vi "[FPGA] DeltaSig Main.vi"() -> ()   [LabVIEW 2015]
doc: "This VI provides a template for customizing a waveform acquisition using delta-sigma based NI C Series analog input smodules."
uses:
  <vilib>/rvi/Emulation/niFpgaGetClockAttributes.vi
  <vilib>/rvi/Emulation/niFpgaSctlEmulationGetInTimedLoop.vi
  <vilib>/rvi/Emulation/niFpgaEmulationReportErrorSimple.vi
  <vilib>/LabVIEW Targets/FPGA/cRIO/shared/nicrio_DsaDataRateApi/_nicrio_9234GetDataRate131.vi
  <vilib>/rvi/Emulation/niFpgaProcessEmulError.vi
  <vilib>/rvi/eio/common/nirviEmuTemplatePropertySet_errors.vi
  <vilib>/rvi/eio/common/nirviEmuTemplateMethod_errors.vi
  <vilib>/rvi/interface/RandomDataEmulation/niFpgaRandomDataHandleErrors.vi
  <vilib>/rvi/Emulation/niFpgaCriticalErrorInLSC.vi
  <vilib>/eio/EIOPropertyNode/EIOPropertyNode.xnode
  <vilib>/LabVIEW Targets/FPGA/cRIO/shared/nicrio_ModuleControls/nicrio_cRIO-9234_DataRatesRing2.ctl
  <vilib>/eio/EIONode/EIONode.xnode
  <vilib>/rvi/DataTransferAndStorage/Container/XNode/niFpgaContainer.xnode
  <vilib>/rvi/interface/RandomDataEmulation/nirviRandomDataFpgaReadWriteTemplate.vi
  <vilib>/rvi/eio/common/nirviEmuTemplatePropertyGet_errors.vi
  <vilib>/rvi/eio/common/nirviEmuTemplatePropertyGet_noerrors.vi
  <vilib>/rvi/eio/common/nirviEmuTemplatePropertySet_noerrors.vi
panel:
  out "oclk freq":u32
  out "oclk div":u32
  out "oclk mult":u32
  in  "data rate (S/s)":u32
  in  "Chan Scale Array":sgl[](array[numeric])=[0.0, 0.0, 0.0, 0.0, 0.0, 0.0, 0.0, 0.0, 0.0, 0.0, 0.0, 0.0, 0.0, 0.0, 0.0, 0.0, 0.0, 0.0, 0.0, 0.0, 0.0, 0.0, 0.0, 0.0, 0.0, 0.0, 0.0, 0.0, 0.0, 0.0, 0.0, 0.0, 0.0, 0.0, 0.0, 0.0, 0.0, 0.0, 0.0, 0.0]
  out "Chan Count":bool
  out "Acq Loop Ticks":u32
  out "FPGA Error":errorcluster
  out "Module Underflow":bool
  out "Finished":bool
  in  "Number of Channels":i32=4
  in  "Samps per Chan [Finite]":i32=5120
  out "First Read":bool
  in  "Acquisition Type":enum16{"Finite Samples", "Continuous Samples"}(ring)
  out "DMA FIFO Full":bool
  in  "stop":bool
  # "Array size fixed at 40\nelements but may be \nexpanded if needed"
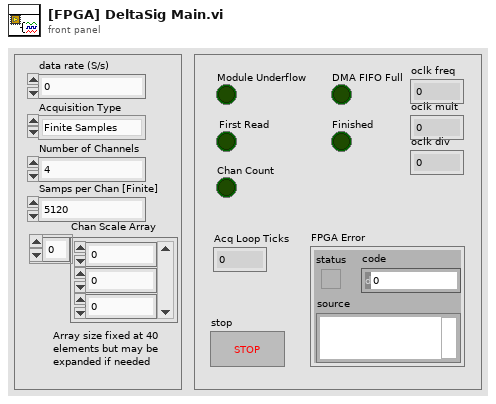
[diagram p1: front panel]
types:
  T1 = typedef "nicrio_cRIO-9234_DataRatesRing2.ctl" = u8
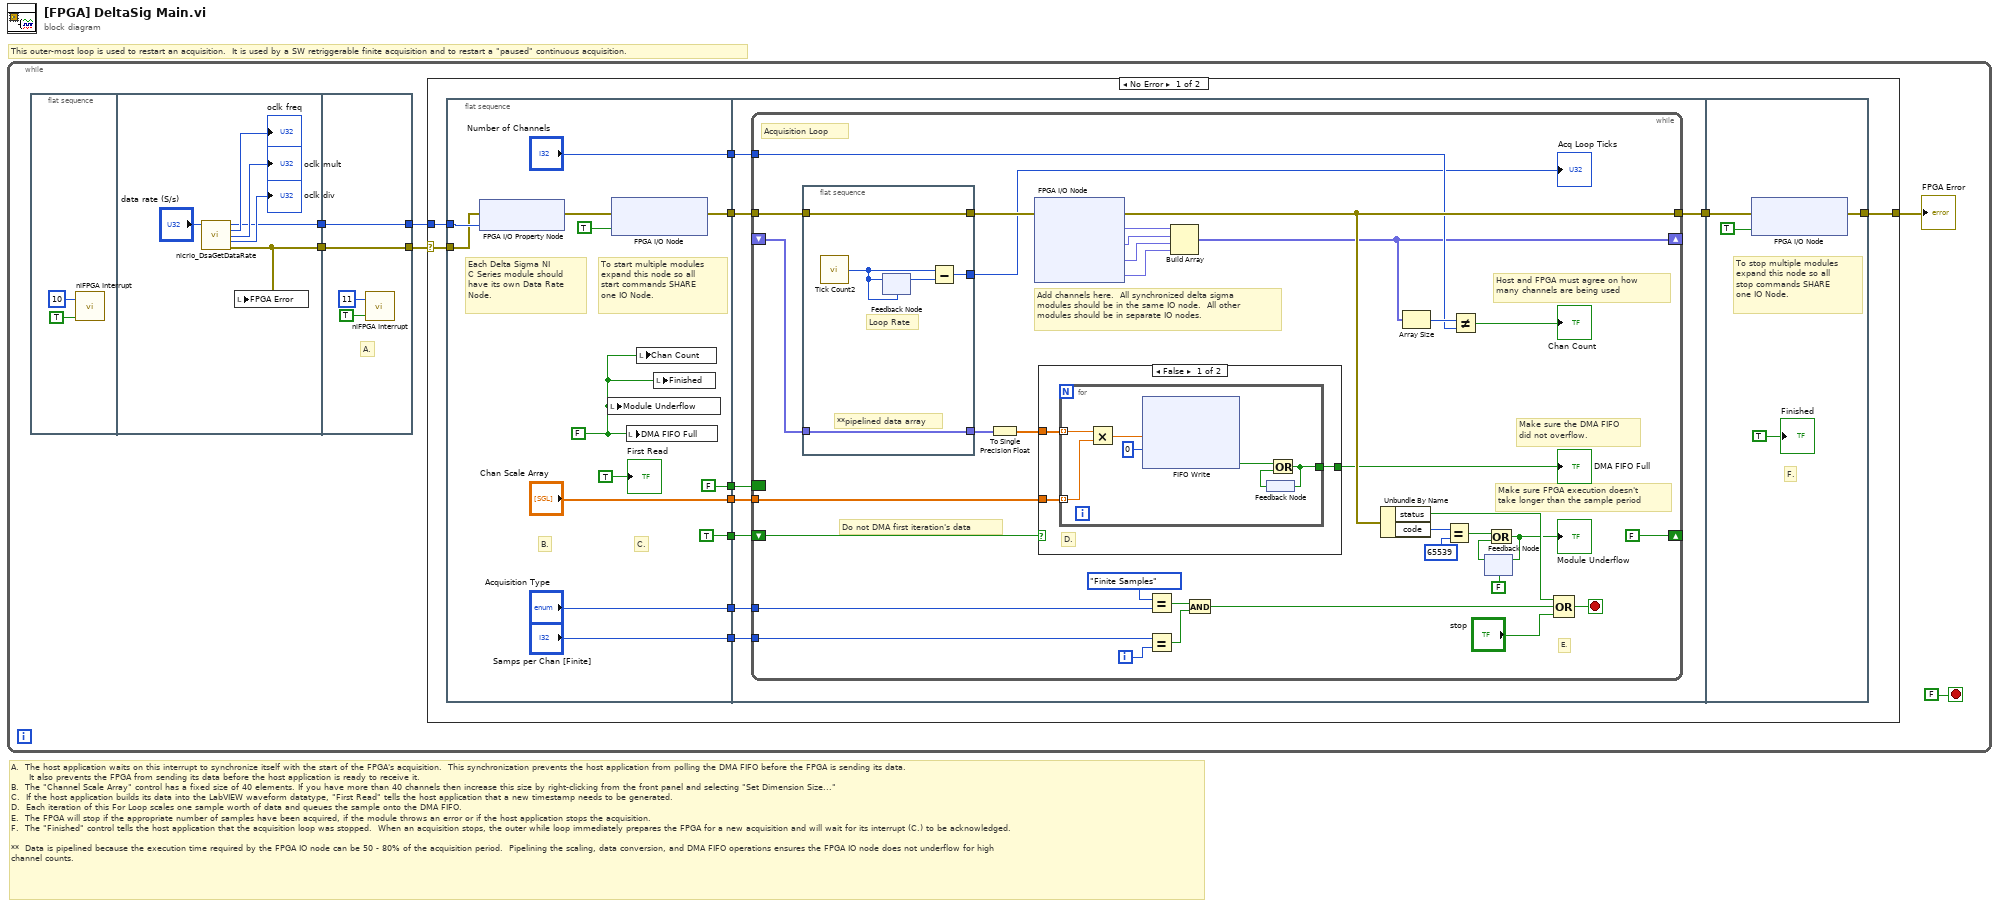
[diagram p0: block diagram]
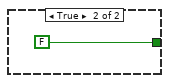
[diagram p2: hidden frame]
diagram:
  # "A.  The host application waits on this interrupt to synchronize itself with the start of the FPGA's acquisition.  This synchronization prevents the host application from polling the DMA FIFO before the FPGA is sending its data.\n      It also prevents the FPGA from sending its data before the host application is ready to receive it.\nB.  The \"Channel Scale Array\" control has a fixed size of 40 elements. If you have more than 40 channels then increase this size by right-clicking from the front panel and selecting \"Set Dimension Size...\"\nC.  If the host application builds its data into the LabVIEW waveform datatype, \"First Read\" tells the host application that a new timestamp needs to be generated.\nD.  Each iteration of this For Loop scales one sample worth of data and queues the sample onto the DMA FIFO.  \nE.  The FPGA will stop if the appropriate number of samples have been acquired, if the module throws an error or if the host application stops the acquisition.  \nF.  The \"Finished\" control tells the host application that the acquisition loop was stopped.  When an acquisition stops, the outer while loop immediately prepares the FPGA for a new acquisition and will wait for its interrupt (C.) to be acknowledged.\n\n**  Data is pipelined because the execution time required by the FPGA IO node can be 50 - 80% of the acquisition period.  Pipelining the scaling, data conversion, and DMA FIFO operations ensures the FPGA IO node does not underflow for high\nchannel counts."
  # "This outer-most loop is used to restart an acquisition.  It is used by a SW retriggerable finite acquisition and to restart a \"paused\" continuous acquisition."
  n1 = while {
    stop <- FALSE stop-if-true
    n2 = flat-sequence {
      tunnel: [w10] -> w2
      tunnel: [w11] -> w1
      tunnel: [w18] -> w3
      tunnel: [w15] -> w4
      tunnel: w2 -> [w15]
      tunnel: w1 -> [w18]
      frame #0 {
        n3 = call <vilib>:"niFPGA Interrupt.vi"("Wait Until Cleared (F)"=TRUE ("Wait Until Cleared"), "IRQ Number (0)"=u8 10 ("IRQ Number")) -> ()  [unwired: 1 in]
      }
      frame #1 {
        n4 = call-poly <vilib>:"nicrio_DsaGetDataRate.vi"("data rate (S/s)"="data rate (S/s)") -> ("data rate"=w11:T1, "oclk freq"=→"oclk freq":u32, "oclk mult"=→"oclk mult":u32, "oclk div"=→"oclk div":u32, "error out"=w10:errorcluster)  [unwired: 10 in]
        n5 = local write "FPGA Error"(w10) -> ()
      }
      frame #2 {
        # "A."
        n6 = call <vilib>:"niFPGA Interrupt.vi"("Wait Until Cleared (F)"=TRUE ("Wait Until Cleared"), "IRQ Number (0)"=u8 11 ("IRQ Number")) -> ()  [unwired: 1 in]
      }
    }
    n7 = case shown="No Error" w4 {
      selector: w4 -> [w19 w106]
      tunnel: [w21 w106] -> w5
      tunnel: w3 -> [w20 _]
      frame No Error {
        n8 = flat-sequence {
          tunnel: [w42] -> w29
          tunnel: ["Chan Scale Array"] -> w28
          tunnel: ["Acquisition Type"] -> w27
          tunnel: ["Samps per Chan [Finite]"] -> w26
          tunnel: ["Number of Channels"] -> w25
          tunnel: [TRUE ("t")] -> w24
          tunnel: [FALSE] -> w23
          tunnel: w20 -> [w31]
          tunnel: w19 -> [w30]
          tunnel: w29 -> [w49]
          tunnel: w28 -> [w48]
          tunnel: w27 -> [w46]
          tunnel: w26 -> [w45]
          tunnel: w25 -> [w50]
          tunnel: w24 -> [w47]
          tunnel: [w44] -> w22
          tunnel: w23 -> [w43]
          tunnel: w22 -> [w103]
          tunnel: [w102] -> w21
          frame #0 {
            w39 = FALSE ("Module Underflow")
            # "To start multiple modules\nexpand this node so all\nstart commands SHARE\none IO Node."
            # "C."
            # "B."
            # "Each Delta Sigma NI \nC Series module should \nhave its own Data Rate \nNode."
            n9 = xnode "FPGA I/O Property Node"("error in"=w30, "Data Rate"=w31) -> ("error out"=w38:errorcluster)  [unwired: 1 in, 1 out]
            n10 = local write "Module Underflow"(w39) -> ()
            n11 = xnode "FPGA I/O Node"("error in"=w38, "Mod1/Start"=TRUE) -> ("error out"=w42:errorcluster)  [unwired: 1 in, 1 out]
            n12 = local write "DMA FIFO Full"(w39) -> ()
            n13 = local write "Chan Count"(w39) -> ()
            n14 = local write "Finished"(w39) -> ()
            "First Read" <- TRUE ("First Read")
          }
          frame #1 {
            n15 = while {
              tunnel: w49 -> [w73]
              tunnel: [w78] -> w44
              tunnel: w46 -> [w80]
              tunnel: w45 -> [w79]
              shift-right: [w53] -> _
              shift-left: _ -> [w66]
              tunnel: w50 -> [w75]
              tunnel: w48 -> [w67]
              shift-right: [FALSE ("t")] -> _
              shift-left: w47 -> [w65]
              border: w43 -> [_]
              i -> [w63]
              stop <- w83 stop-if-true
              # "Add channels here.  All synchronized delta sigma\nmodules should be in the same IO node.  All other\nmodules should be in separate IO nodes."
              # "Do not DMA first iteration's data"
              # "Acquisition Loop"
              # "E."
              # "Host and FPGA must agree on how \nmany channels are being used"
              # "Make sure the DMA FIFO\ndid not overflow."
              # "Make sure FPGA execution doesn't\ntake longer than the sample period"
              n16 = flat-sequence {
                tunnel: [w101] -> w72
                tunnel: w73 -> [w101]
                tunnel: [w98] -> w71
                tunnel: w66 -> [w97]
                tunnel: [w97] -> w52
                frame #0 {
                  # "**pipelined data array"
                  # "Loop Rate"
                  n17 = call "Tick Count2"() -> ("Tick Count(Ticks)"=w100:u32)
                  n18 = feedback-in #1(w100) -> ()
                  n19 = feedback #1(w100) -> (w99:u32)
                  n20 = Subtract(x=w100, y=w99) -> (x-y=w98:u32)
                }
              }
              n21 = To Single Precision Float(number=w52) -> (single precision float=w51:sgl[])
              n22 = xnode "FPGA I/O Node"("error in"=w72) -> ("error out"=w78:errorcluster, "Mod1/AI0"=w70:fxp<+/-,24,4>, "Mod1/AI1"=w62:fxp<+/-,24,4>, "Mod1/AI2"=w69:fxp<+/-,24,4>, "Mod1/AI3"=w68:fxp<+/-,24,4>)  [unwired: 4 in, 4 out]
              n23 = case shown="False" w65 {
                tunnel: [w88 FALSE] -> w77
                tunnel: w67 -> [w87 _]
                tunnel: w51 -> [w86 _]
                frame False {
                  # "D."
                  n24 = for {
                    tunnel: [w93] -> w88
                    tunnel: w86 -> [w91] mode=indexing
                    tunnel: w87 -> [w90] mode=indexing
                    n25 = Multiply(x=w91, y=w90) -> (x*y=w89:sgl)
                    n26 = xnode ("FIFO Write")("Element"=w89, "Timeout"=0) -> ("Timed Out?"=w95:bool)  [unwired: 1 in, 1 out]
                    n27 = feedback #2() -> (w94:bool)
                    n28 = Or(x=w95, y=w94) -> (x .or. y?=w93:bool)
                    n29 = feedback-in #2(w93) -> ()
                  }
                }
                frame True {
                }
              }
              "DMA FIFO Full" <- w77
              n30 = Equal?(x=enum16{"Finite Samples", "Continuous Samples"}."Finite Samples" ("y"), y=w80) -> (x = y?=w56:bool)
              n31 = Equal?(x=w79, y=w63) -> (x = y?=w55:bool)
              n32 = Build Array(w70, w62, w69, w68) -> (w53:fxp<+/-,24,4>[])
              n33 = And(x=w56, y=w55) -> (x .and. y?=w54:bool)
              n34 = Unbundle By Name(w78) -> ("status"=w61:bool, "code"=w81:i32)
              n35 = Array Size(array=w53) -> (size(s)=w76:i32)
              n36 = Equal?(x=w81, y=65539) -> (x = y?=w58:bool)
              n37 = Not Equal?(x=w76, y=w75) -> (x != y?=→"Chan Count":bool)
              n38 = feedback #3(FALSE) -> (w60:bool)
              n39 = Or(x=w58, y=w60) -> (x .or. y?=w57:bool)
              "Module Underflow" <- w57
              n40 = feedback-in #3(w57) -> ()
              n41 = Compound Arithmetic op=OR(w61, w54, "stop") -> (w83:bool)
              "Acq Loop Ticks" <- w71
            }
          }
          frame #2 {
            # "To stop multiple modules\nexpand this node so all\nstop commands SHARE\none IO Node."
            # "F."
            n42 = xnode "FPGA I/O Node"("error in"=w103, "Mod1/Stop"=TRUE) -> ("error out"=w102:errorcluster)  [unwired: 1 in, 1 out]
            "Finished" <- TRUE ("Finished")
          }
        }
      }
      frame Error {
      }
    }
    "FPGA Error" <- w5
  }
